vi "Get Position History.vi"(8 "Error In":errorcluster, 11 "Pixel In":refnum<class "Pixel.lvclass">) -> (0 "Error Out":errorcluster, 2 "Positions History":T1[](array[typedef]), 3 "Pixel Out":refnum<class "Pixel.lvclass">)   [LabVIEW 2019, in "Pixel.lvclass"]
uses:
  Pixel.lvclass
  Display Utilities/Public/Controls/2D Coordenates.ctl
  Display Utilities/Display Utilities.lvlib
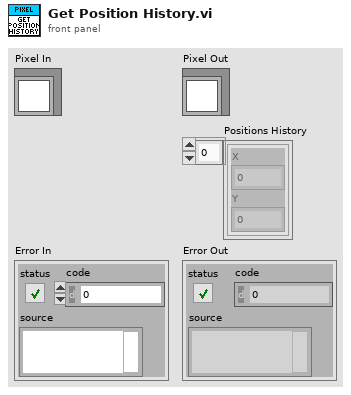
[diagram p1: front panel]
types:
  T1 = typedef "Display Utilities.lvlib/2D Coordenates.ctl" = cluster{"X":i32, "Y":i32}
  T2 = typedef "Pixel.lvclass/Data.ctl" = cluster{"Trace":i32, "Positions History":T3[]}
  T3 = typedef "Display Element.lvclass/Vector.ctl" = cluster{"X":i32, "Y":i32}
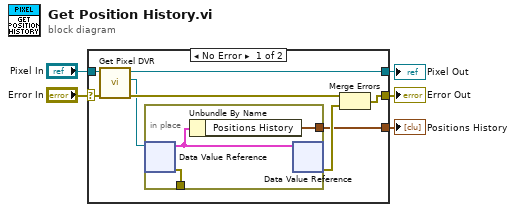
[diagram p0: block diagram]
diagram:
  n1 = case shown="No Error" "Error In" {
    selector: "Error In" -> [w9 w17]
    tunnel: [w11 w17] -> w4
    tunnel: [w6 w18] -> w1
    tunnel: "Pixel In" -> [w10 w18]
    tunnel: [w12 _] -> w2
    frame No Error {
      n2 = call "Get Pixel DVR.vi"("Error In"=w9, "Pixel In"=w10) -> ("Error Out"=w8:errorcluster, "DVR"=w7:refnum<data-value>, "Pixel Out"=w6:refnum<class "Pixel.lvclass">)  [unwired: 7 in]
      n3 = in-place {
        in-place-border: [w14] -> w12
        in-place-border: [w16] -> _
        n4 = in-place-dvr #1(w7) -> (w15:T2, w16:errorcluster)
        n5 = Unbundle By Name(w15) -> ("Positions History"=w14:T3[])
        n6 = in-place-dvr #1(w15) -> (w13:errorcluster)  [unwired: 1 out]
      }
      n7 = Merge Errors(w8, w13) -> (w11:errorcluster)
    }
    frame Error {
    }
  }
  "Pixel Out" <- w1
  "Error Out" <- w4
  "Positions History" <- w2
